vi "fpga_Get Position.vi"(0 "tach input":fxp<+/-,24,3>, 1 "Interpolation factor":u16=64, 5 "Fnom":T1 items=["Fnom=50Hz", "Fnom=60Hz"], 9 "input valid":bool, 12 "ready for output":bool) -> (4 "resample position [U64.16]":fxp<+,64,16> format="%.53g", 6 "stepsize [U64.8]":fxp<+,64,8>, 8 "frequency":fxp<+,32,8> format="%.27g", 10 "output valid":bool, 14 "Ready for input":bool, 15 "resampling valid":bool)   [LabVIEW 2015, in "NI_EP_Resample_FPGA.lvlib"]
uses:
  <vilib>/addons/Electrical Power/PQ/Resampling/NI_EP_Resample_FPGA.lvlib
  <vilib>/addons/Electrical Power/PQ/Resampling/FPGA/subVIs/fpga_Typedef Fnom.ctl
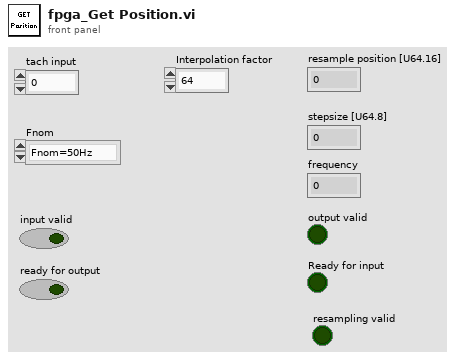
[diagram p1: front panel]
types:
  T1 = typedef "NI_EP_Resample_FPGA.lvlib/fpga_Typedef Fnom.ctl" = u8
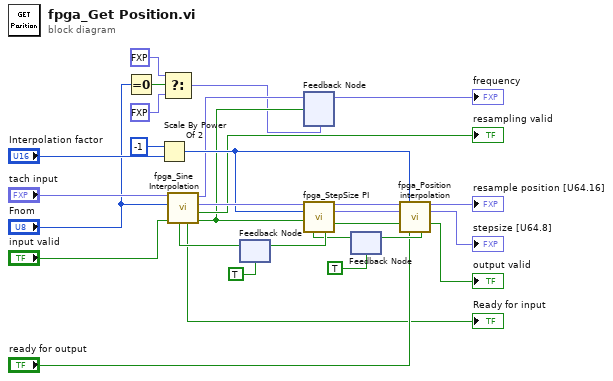
[diagram p0: block diagram]
diagram:
  n1 = Equal To 0?(x="Fnom") -> (x = 0?=w4:bool)
  n2 = Scale By Power Of 2(n=-1, x="Interpolation factor") -> (x*2^n=w12:u16)
  n3 = Select(t=fxp<+,32,8> 50.0 ("frequency"), s=w4, f=fxp<+,32,8> 60.0 ("frequency")) -> (s? t:f=w1:fxp<+,32,8>)
  n4 = feedback #1(TRUE ("ready for input")) -> (w14:bool)
  n5 = call <vilib>:"fpga_Sine Interpolation.vi"("ready for output"=w14, "input valid"="input valid", "Fnom"="Fnom", "tach input"="tach input") -> ("output valid"=w7:bool, "resampling valid"=→"resampling valid":bool, "crossing"=w17:fxp<+,32,16>, "frequency"=w10:fxp<+,32,8>, "ready for input"=→"Ready for input":bool)  [unwired: 3 in]
  n6 = feedback-in #2(w10, w7) -> ()
  n7 = feedback #2(w1) -> (→"frequency":fxp<+,32,8>)
  n8 = feedback #3(TRUE ("ready for input")) -> (w20:bool)
  n9 = call <vilib>:"fpga_StepSize PI.vi"("Crossing U[32.16]"=w17, "interpolation factor"=w12, "input valid"=w7, "ready for output"=w20) -> ("Crossing[U64.16]"=w24:fxp<+,64,16>, "Stepsize[U64.8]"=w23:fxp<+,64,8>, "output valid"=w22:bool, "ready for input"=w26:bool)  [unwired: 8 in]
  n10 = feedback-in #1(w26) -> ()
  n11 = call <vilib>:"fpga_Position interpolation.vi"("Crossing[U64.16]"=w24, "Interpolation factor"=w12, "Stepsize[U64.8]"=w23, "input valid"=w22, "ready for output"="ready for output") -> ("resample position [U64.16]"=→"resample position [U64.16]":fxp<+,64,16>, "stepsize [U64.8]"=→"stepsize [U64.8]":fxp<+,64,8>, "output valid"=→"output valid":bool, "ready for input"=w21:bool)  [unwired: 1 in, 6 out]
  n12 = feedback-in #3(w21) -> ()
